vi "Write Path Commands.vi"(8 "error in (no error)":errorcluster, 10 "Path Commands":refnum<class "PathCommands.lvclass">[](array[class]), 11 "Path in":refnum<class "Path.lvclass">) -> (0 "error out":errorcluster, 3 "Path out":refnum<class "Path.lvclass">)   [LabVIEW 2019, in "Path.lvclass"]
uses:
  Path.lvclass
  PathCommands/PathCommands.lvclass
  Path.lvclass/Path.ctl
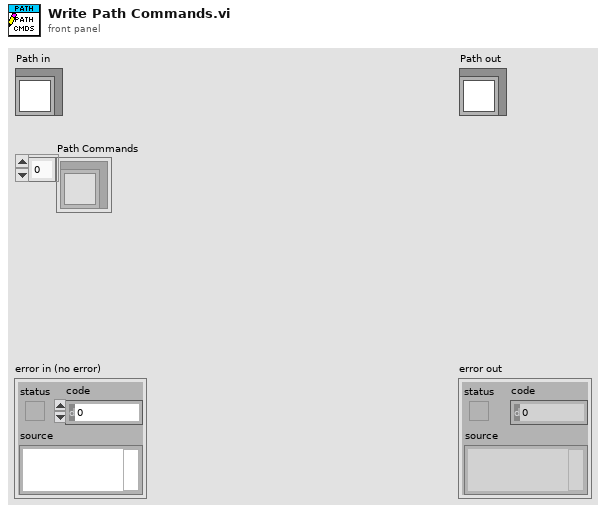
[diagram p1: front panel]
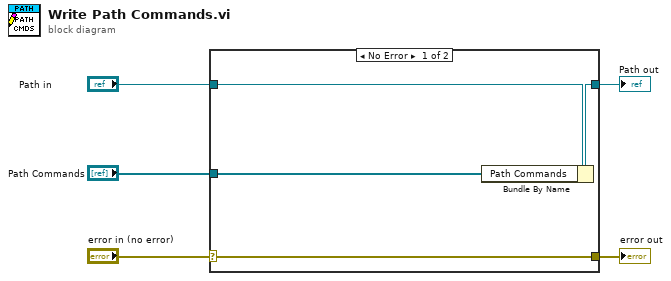
[diagram p0: block diagram]
diagram:
  n1 = case shown="No Error" "error in (no error)" {
    selector: "error in (no error)" -> [w9 w10]
    tunnel: [w9 w10] -> w4
    tunnel: [w7 w11] -> w2
    tunnel: "Path in" -> [w8 w11]
    tunnel: "Path Commands" -> [w6 _]
    frame No Error {
      n2 = Bundle By Name(cluster=w8, "Path Commands"=w6) -> (w7:refnum<class "Path.lvclass">)
    }
    frame Error {
    }
  }
  "error out" <- w4
  "Path out" <- w2
